vi "as. licznik binarny.vi"(10 "CP":bool) -> (0 "iloœæ zliczeñ":u32, 3 "Tablica zliczeñ":bool[](array[boolean]))   [LabVIEW 2020]
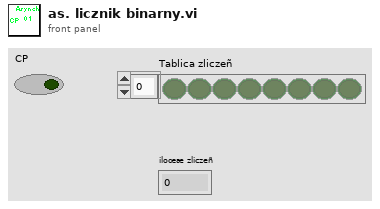
[diagram p1: front panel]
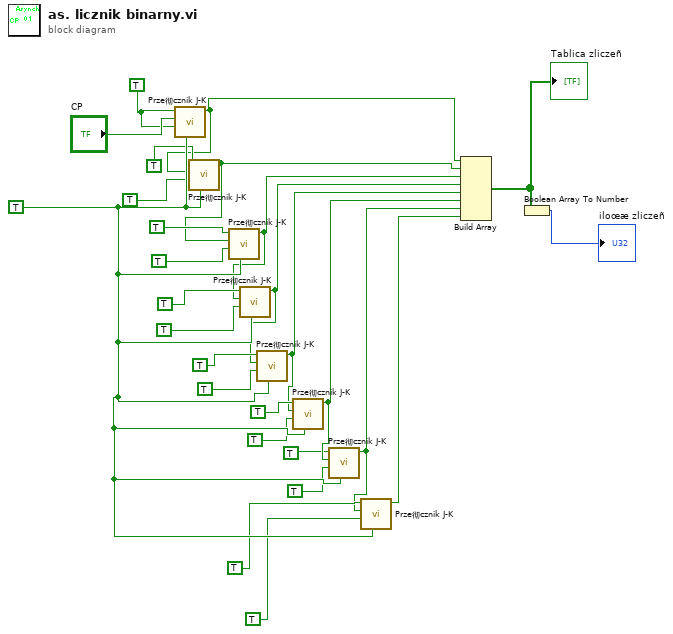
[diagram p0: block diagram]
diagram:
  w27 = TRUE ("R")
  w3 = TRUE ("J")
  n1 = call "Prze彻cznik J-K.vi"("R"=w27, "K"=w3, "C"="CP", "J"=w3) -> ("Q"=w5:bool)  [unwired: 6 in, 1 out]
  n2 = call "Prze彻cznik J-K.vi"("R"=w27, "K"=TRUE ("J"), "C"=w5, "J"=TRUE ("K")) -> ("Q"=w8:bool)  [unwired: 6 in, 1 out]
  n3 = call "Prze彻cznik J-K.vi"("R"=w27, "K"=TRUE ("J"), "C"=w8, "J"=TRUE ("K")) -> ("Q"=w11:bool)  [unwired: 6 in, 1 out]
  n4 = call "Prze彻cznik J-K.vi"("R"=w27, "K"=TRUE, "C"=w11, "J"=TRUE ("K")) -> ("Q"=w14:bool)  [unwired: 6 in, 1 out]
  n5 = call "Prze彻cznik J-K.vi"("R"=w27, "K"=TRUE ("J"), "C"=w14, "J"=TRUE ("K")) -> ("Q"=w17:bool)  [unwired: 6 in, 1 out]
  n6 = call "Prze彻cznik J-K.vi"("R"=w27, "K"=TRUE ("J"), "C"=w17, "J"=TRUE ("K")) -> ("Q"=w22:bool)  [unwired: 6 in, 1 out]
  n7 = call "Prze彻cznik J-K.vi"("R"=w27, "K"=TRUE ("J"), "C"=w22, "J"=TRUE ("K")) -> ("Q"=w23:bool)  [unwired: 6 in, 1 out]
  n8 = call "Prze彻cznik J-K.vi"("R"=w27, "K"=TRUE ("J"), "C"=w23, "J"=TRUE ("K")) -> ("Q"=w24:bool)  [unwired: 6 in, 1 out]
  n9 = Build Array(w5, w8, w11, w14, w17, w22, w23, w24) -> (w1:bool[])
  "Tablica zliczeñ" <- w1
  n10 = Boolean Array To Number(Boolean array=w1) -> (number=→"iloœæ zliczeñ":u32)
